vi "GenCodeScripts-ReplaceContent.vi"(8 "error in (no error)":errorcluster, 9 "template":path, 10 "Terms":T2, 11 "Diagram":T1) -> (0 "error out":errorcluster, 2 "Terms out":T2, 3 "Diagram out":T1)   [LabVIEW 2017, in "ReadTag.xnode"]
doc: "Read Tag XNode script that opens the code template and replaces its placeholder content with the generated terms."
uses:
  ReadTag.xnode
  <vilib>/XNodeSupport/XNodeTopLevelDiagramRef.ctl
  <vilib>/XNodeSupport/XNodeTermIDPairs.ctl
  <vilib>/XNodeSupport/XNodeTermIDPair.ctl
  <vilib>/XNodeSupport/XNodeTermRef.ctl
  <vilib>/XNodeSupport/XNodeString.ctl
  <vilib>/Utility/miscctls.llb/LVPositionTypeDef.ctl
  <vilib>/XNodeSupport/NI_XNodeSupport.lvlib
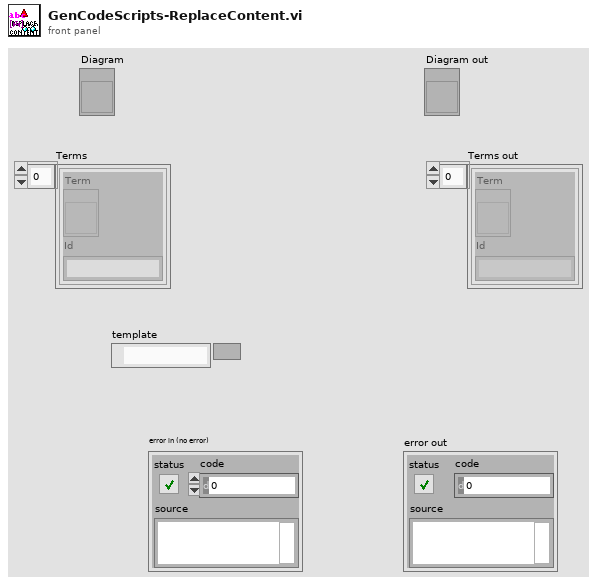
[diagram p1: front panel]
types:
  T1 = typedef "NI_XNodeSupport.lvlib/XNodeTopLevelDiagramRef.ctl" = refnum<vi>
  T2 = typedef "NI_XNodeSupport.lvlib/XNodeTermIDPairs.ctl" = T3[]
  T3 = typedef "NI_XNodeSupport.lvlib/XNodeTermIDPair.ctl" = cluster{"Term":T4, "Id":T5}
  T4 = typedef "NI_XNodeSupport.lvlib/XNodeTermRef.ctl" = refnum<vi>
  T5 = typedef "NI_XNodeSupport.lvlib/XNodeString.ctl" = string
  T6 = typedef "LVPositionTypeDef.ctl" = cluster{"Left":i32, "Top":i32}
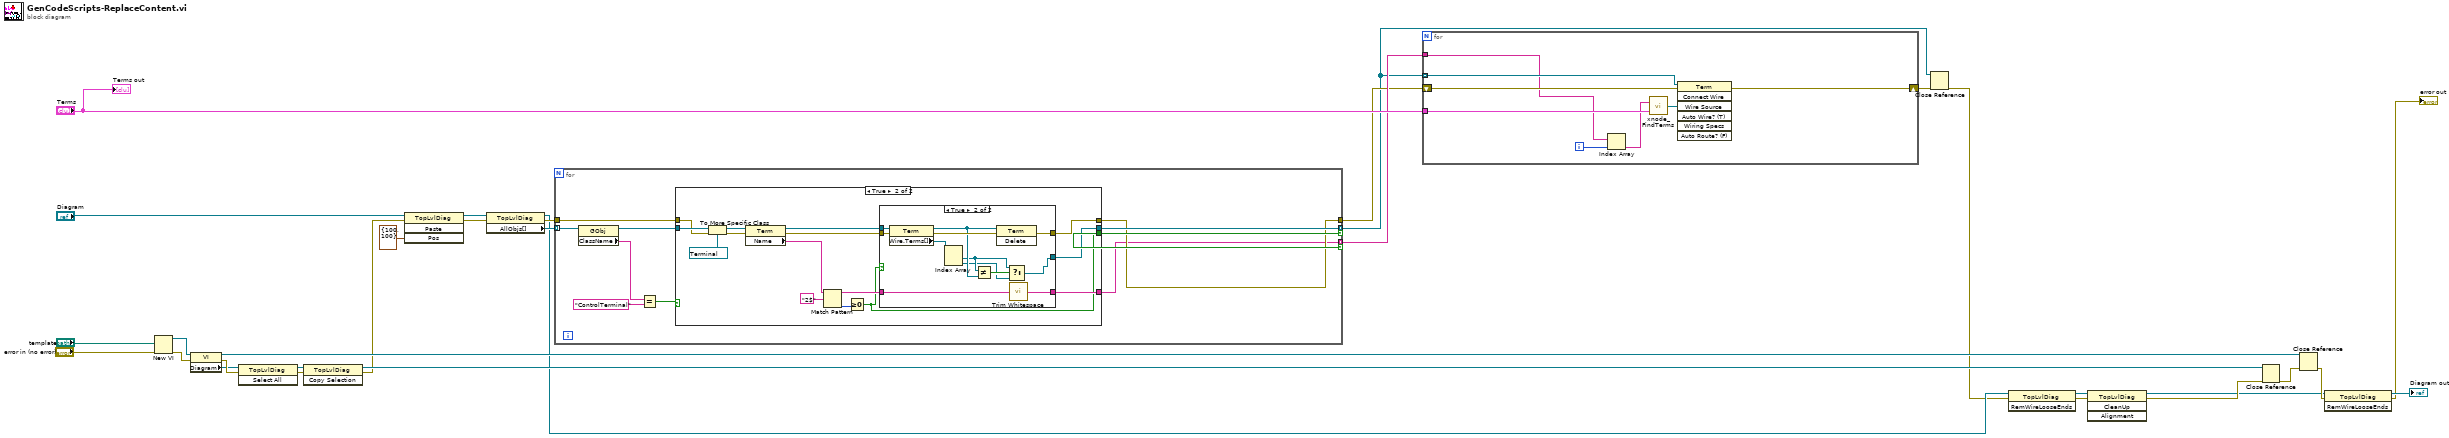
[diagram p0: block diagram]
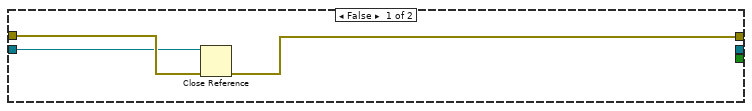
[diagram p2: hidden frame]
diagram:
  n1 = New VI(8:"error in (no error)", 10:"template") -> (0:w18:errorcluster, 3:w17:refnum<vi>)  [unwired: 5 in]
  n2 = property class="VI"(reference=w17, error in=w18) -> (reference out=w26:refnum<vi>, error out=w29:errorcluster, "Diagram"=w19:refnum<vi>)
  n3 = invoke class="TopLvlDiag" method="Select All"(reference=w19, error in=w29) -> (reference out=w20:refnum<vi>, error out=w21:errorcluster)  [unwired: 1 in, 1 out]
  n4 = invoke class="TopLvlDiag" method="Copy Selection"(reference=w20, error in=w21) -> (reference out=w23:refnum<vi>, error out=w22:errorcluster)  [unwired: 1 in, 1 out]
  n5 = invoke class="TopLvlDiag" method="Paste"(reference="Diagram", error in=w22, "Pos"=T6 {"Left"=100, "Top"=100} ("Position")) -> (reference out=w27:T1, error out=w28:errorcluster)  [unwired: 1 in, 2 out]
  n6 = property class="TopLvlDiag"(reference=w27, error in=w28) -> (reference out=w11:T1, error out=w30:errorcluster, "AllObjs[]"=w13:refnum<vi>[])
  n7 = for {
    tunnel: w13 -> [w39] mode=indexing
    tunnel: [w33] -> w14 mode=indexing if=w42
    tunnel: [w41] -> w6 mode=indexing if=w42
    tunnel: w30 -> [w40]
    tunnel: [w34] -> w12
    n8 = property class="GObj"(reference=w39) -> (reference out=w36:refnum<vi>, "ClassName"=w38:string)  [unwired: 1 in, 1 out]
    n9 = Equal?(x=w38, y="ControlTerminal") -> (x = y?=w35:bool)
    n10 = case shown="True" w35 {
      tunnel: [w44 w52] -> w34
      tunnel: [_ w46] -> w42
      tunnel: [_ w56] -> w33
      tunnel: [_ w49] -> w41
      tunnel: w40 -> [w45 w48]
      tunnel: w36 -> [w43 w55]
      frame False {
        n11 = Close Reference(reference=w43, error in (no error)=w45) -> (error out=w44:errorcluster)
      }
      frame True {
        n12 = To More Specific Class(target class=refnum<vi> refnum ("reference"), reference=w55, error in=w48) -> (specific class reference=w51:refnum<vi>, error out=w47:errorcluster)
        n13 = property class="Term"(reference=w51, error in=w47) -> (reference out=w54:refnum<vi>, error out=w53:errorcluster, "Name"=w60:string)
        n14 = Match Pattern(string=w60, regular expression="2$") -> (before substring=w59:string, offset past match=w57:i32)  [unwired: 1 in, 2 out]
        n15 = Greater Or Equal To 0?(x=w57) -> (x >= 0?=w46:bool)
        n16 = case shown="True" w46 {
          tunnel: w59 -> [_ w73]
          tunnel: [_ w72] -> w56
          tunnel: w54 -> [_ w70]
          tunnel: w53 -> [w61 w69]
          tunnel: [w61 w71] -> w52
          tunnel: [_ w62] -> w49
          frame False {
          }
          frame True {
            n17 = property class="Term"(reference=w70, error in=w69) -> (reference out=w66:refnum<vi>, error out=w68:errorcluster, "Wire.Terms[]"=w67:refnum<vi>[])
            n18 = Index Array(array=w67) -> (element #1=w64:refnum<vi>, element #2=w63:refnum<vi>)  [unwired: 2 in]
            n19 = Not Equal?(x=w64, y=w66) -> (x != y?=w65:bool)
            n20 = invoke class="Term" method="Delete"(reference=w66, error in=w68) -> (error out=w71:errorcluster)  [unwired: 1 in, 2 out]
            n21 = Select(t=w64, s=w65, f=w63) -> (s? t:f=w62:refnum<vi>)
            n22 = call <vilib>:"Trim Whitespace.vi"("string"=w73) -> ("trimmed string"=w72:string)  [unwired: 1 in]
          }
        }
      }
    }
  }
  n23 = for {
    tunnel: "Terms" -> [w81]
    tunnel: w6 -> [w80] mode=indexing
    tunnel: w14 -> [w78]
    shift-right: [w74] -> w31
    shift-left: w12 -> [w79]
    i -> [w76]
    n24 = Index Array(array=w78, index=w76) -> (element=w77:string)
    n25 = call "xnode_FindTerms.vi"("Terms"=w81, "String"=w77) -> ("Terminal"=w75:T4)
    n26 = invoke class="Term" method="Connect Wire"(reference=w80, error in=w79, "Wire Source"=w75) -> (error out=w74:errorcluster)  [unwired: 4 in, 6 out]
  }
  n27 = Close Reference(reference=w6, error in (no error)=w31) -> (error out=w7:errorcluster)
  n28 = invoke class="TopLvlDiag" method="RemWireLooseEnds"(reference=w11, error in=w7) -> (reference out=w8:T1, error out=w10:errorcluster)  [unwired: 1 in, 1 out]
  n29 = invoke class="TopLvlDiag" method="CleanUp"(reference=w8, error in=w10) -> (reference out=w4:T1, error out=w9:errorcluster)  [unwired: 2 in, 2 out]
  n30 = Close Reference(reference=w23, error in (no error)=w9) -> (error out=w24:errorcluster)
  n31 = Close Reference(reference=w26, error in (no error)=w24) -> (error out=w5:errorcluster)
  n32 = invoke class="TopLvlDiag" method="RemWireLooseEnds"(reference=w4, error in=w5) -> (reference out=→"Diagram out":T1, error out=→"error out":errorcluster)  [unwired: 1 in, 1 out]
  "Terms out" <- "Terms"
